vi "TC560-Read Command Data.vi"(8 "error in":errorcluster) -> (0 "error out":errorcluster, 3 "Configuration":T1={"Connection Setting"={"VISA Resource Name"="", "Baud Rate"=9600, "Parity"=0, "Flow Control"=0}, "Wait For Read"=0} {"Connection Setting"."Flow Control" items=["None", "XON/XOFF", "RTS/CTS", "XON/XOFF & RTS/CTS", "DTR/DSR", "XON/XOFF & DTR/DSR"]; "Connection Setting"."Parity" items=["None", "Odd", "Even", "Mark", "Space"]; "Connection Setting"."Baud Rate" items=["2400"=2400, "4800"=4800, "9600"=9600]})   [LabVIEW 2018]
uses:
  Data Def/TC560-Configuration.ctl
  Data Def/TC560-Connection Setting.ctl
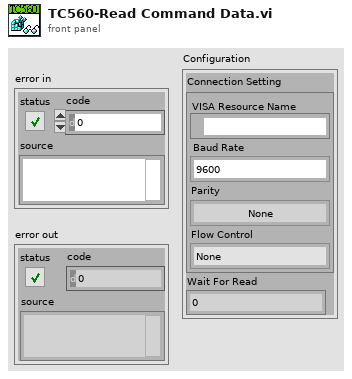
[diagram p1: front panel]
types:
  T1 = typedef "TC560-Configuration.ctl" = cluster{"Connection Setting":T2, "Wait For Read":u32}
  T2 = typedef "TC560-Connection Setting.ctl" = cluster{"VISA Resource Name":refnum<visa-resource-name>, "Baud Rate":u32, "Parity":u16, "Flow Control":u16}
  T3 = enum16{"open", "replace", "create", "open or create", "replace or create", "replace or create with confirmation"}
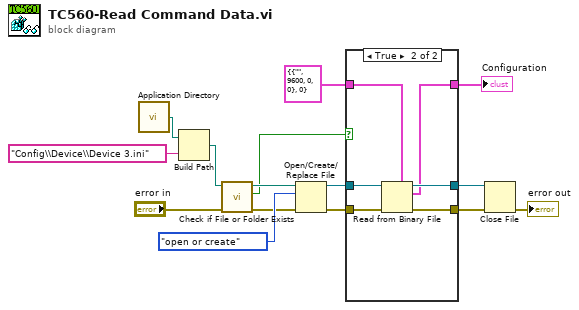
[diagram p0: block diagram]
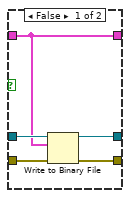
[diagram p2: hidden frame]
diagram:
  n1 = call <vilib>:"Application Directory.vi"() -> ("Application Directory"=w7:path)
  n2 = Build Path(base path=w7, name or relative path="Config\\Device\\Device 3.ini") -> (appended path=w5:path)
  n3 = call <vilib>:"Check if File or Folder Exists.vi"("error in (no error)"="error in", "path"=w5) -> ("error out"=w14:errorcluster, "file or folder exists?"=w11:bool, "dup path"=w13:path)  [unwired: 7 in]
  n4 = Open/Create/Replace File(file path (use dialog)=w13, error in=w14, operation (0:open)=T3."open or create") -> (refnum out=w10:refnum<file>, error out=w12:errorcluster)  [unwired: 3 in, 1 out]
  n5 = case shown="True" w11 {
    tunnel: w12 -> [w20 w26]
    tunnel: w10 -> [w19 w25]
    tunnel: T1 {"Connection Setting"={"VISA Resource Name"="", "Baud Rate"=9600, "Parity"=0, "Flow Control"=0}, "Wait For Read"=0} ("Configuration") -> [w16 w24]
    tunnel: [w18 w23] -> w8
    tunnel: [w17 w22] -> w9
    tunnel: [w16 w21] -> w1
    frame False {
      n6 = Write to Binary File(file (use dialog)=w19, data=w16, error in=w20) -> (refnum out=w18:refnum<file>, error out=w17:errorcluster)  [unwired: 3 in, 1 out]
    }
    frame True {
      n7 = Read from Binary File(5:w24, 8:w26, 11:w25) -> (0:w22:errorcluster, 2:w21:T1, 3:w23:refnum<file>)  [unwired: 3 in, 1 out]
    }
  }
  "Configuration" <- w1
  n8 = Close File(refnum=w8, error in=w9) -> (error out=→"error out":errorcluster)  [unwired: 1 out]
